vi "Day 5.2 - .vi"(11 "input":string[](array[string])) -> (3 "output":string)   [LabVIEW 2021]
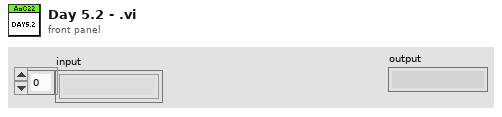
[diagram p1: front panel]
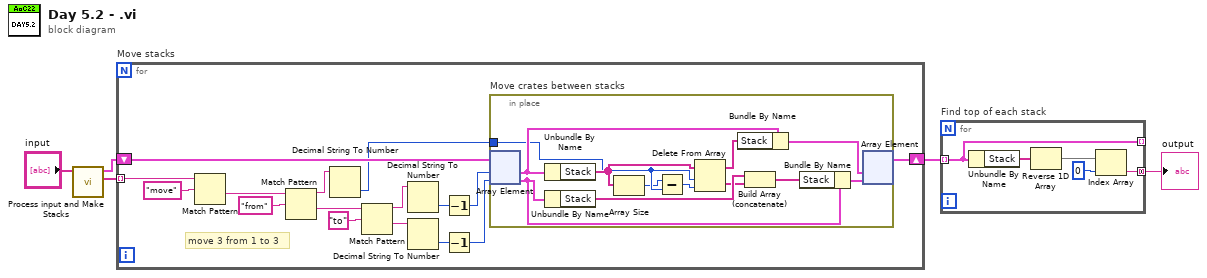
[diagram p0: block diagram]
diagram:
  n1 = call "Process input and Make Stacks.vi"("input"="input") -> ("Moves"=w5:string[], "Stacks"=w4:cluster{"Label":string, "Stack":string[]}[])  [unwired: 9 in]
  n2 = for "Move stacks" {
    tunnel: w5 -> [w21] mode=indexing
    shift-right: [w9] -> w3
    shift-left: w4 -> [w12]
    # "move 3 from 1 to 3"
    n3 = Match Pattern(string=w21, regular expression="move") -> (after substring=w19:string)  [unwired: 1 in, 3 out]
    n4 = Match Pattern(string=w19, regular expression="from") -> (before substring=w15:string, after substring=w17:string)  [unwired: 1 in, 2 out]
    n5 = Decimal String To Number(string=w15) -> (number=w6:i32)  [unwired: 2 in, 1 out]
    n6 = Match Pattern(string=w17, regular expression="to") -> (before substring=w14:string, after substring=w13:string)  [unwired: 1 in, 2 out]
    n7 = Decimal String To Number(string=w14) -> (number=w11:i32)  [unwired: 2 in, 1 out]
    n8 = Decimal String To Number(string=w13) -> (number=w10:i32)  [unwired: 2 in, 1 out]
    n9 = Decrement(x=w11) -> (x-1=w8:i32)
    n10 = Decrement(x=w10) -> (x-1=w7:i32)
    n11 = in-place "Move crates between stacks" {
      in-place-border: w6 -> [w23]
      n12 = in-place-array #1(w12, w8, w7) -> (w32:cluster{"Label":string, "Stack":string[]}, w30:cluster{"Label":string, "Stack":string[]})
      n13 = Unbundle By Name(w32) -> ("Stack"=w29:string[])
      n14 = Unbundle By Name(w30) -> ("Stack"=w26:string[])
      n15 = Array Size(array=w29) -> (size(s)=w22:i32)
      n16 = Subtract(x=w22, y=w23) -> (x-y=w28:i32)
      n17 = Delete From Array(array=w29, length=w23, index=w28) -> (deleted portion=w25:string[], array with subset deleted=w27:string[])
      n18 = Bundle By Name(cluster=w32, "Stack"=w27) -> (w33:cluster{"Label":string, "Stack":string[]})
      n19 = Build Array (concatenate)(w26, w25) -> (w24:string[])
      n20 = Bundle By Name(cluster=w30, "Stack"=w24) -> (w31:cluster{"Label":string, "Stack":string[]})
      n21 = in-place-array #1(w33, w31) -> (w9:cluster{"Label":string, "Stack":string[]}[])  [unwired: 2 out]
    }
  }
  n22 = for "Find top of each stack" {
    tunnel: [w34] -> _ mode=indexing
    tunnel: [w35] -> w1 mode=concatenating
    tunnel: w3 -> [w34] mode=indexing
    n23 = Unbundle By Name(w34) -> ("Stack"=w38:string[])
    n24 = Reverse 1D Array(array=w38) -> (reversed array=w37:string[])
    n25 = Index Array(array=w37, index=0) -> (element=w35:string)
  }
  "output" <- w1
